vi "Add PV - I32 Array.vi"(5 "is read only? (F)":bool, 6 "initial timestamp":timestamp, 7 "PV name":string, 8 "error in (no error)":errorcluster, 9 "fields":T1, 10 "initial value":i32[](array[numeric]), 11 "Server in":refnum<class "Server.lvclass">) -> (0 "error out":errorcluster, 3 "Server out":refnum<class "Server.lvclass">)   [LabVIEW 2020, in "PV Access.lvlib" / "PVA Server.lvlib" / "Server.lvclass"]
uses:
  Server.lvclass
  PV Data/Value Fields.ctl
  PV Data/NT Scalar (Numeric)/NT Scalar (Numeric).lvclass
  C:/Users/eyw68381/source/repos/pvaccess-labview/labview/source/PV Data/Base/Base.lvclass
  PV Data/NT Scalar (Numeric)/Create - I32 Array.vi
  Source/Source.lvclass
  PV Data/PV Data.lvlib
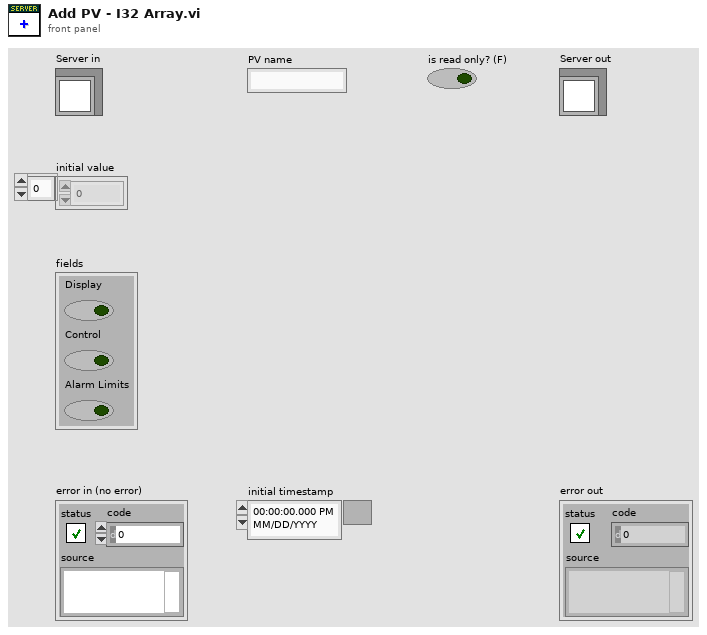
[diagram p1: front panel]
types:
  T1 = typedef "PV Access.lvlib/PV Data.lvlib/Value Fields.ctl" = cluster{"Display":bool, "Control":bool, "Alarm Limits":bool}
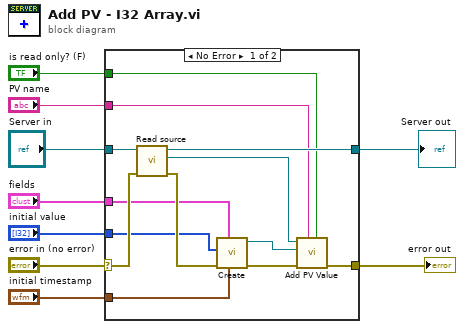
[diagram p0: block diagram]
diagram:
  n1 = case shown="No Error" "error in (no error)" {
    selector: "error in (no error)" -> [w18 w24]
    tunnel: [w17 w24] -> w8
    tunnel: [w21 w23] -> w6
    tunnel: "Server in" -> [w22 w23]
    tunnel: "PV name" -> [w19 _]
    tunnel: "initial value" -> [w13 _]
    tunnel: "fields" -> [w12 _]
    tunnel: "initial timestamp" -> [w11 _]
    tunnel: "is read only? (F)" -> [w10 _]
    frame No Error {
      n2 = call "Read source.vi"("error in (no error)"=w18, "Server in"=w22) -> ("error out"=w16:errorcluster, "Source"=w20:refnum<class "Source.lvclass">, "Server out"=w21:refnum<class "Server.lvclass">)  [unwired: 7 in]
      n3 = call-poly "Create.vi"("timestamp"=w11, "fields"=w12, "error in (no error)"=w16, "value"=w13) -> ("error out"=w15:errorcluster, "NT Scalar (Numeric) out"=w14:refnum<class "NT Scalar (Numeric).lvclass">)  [unwired: 6 in]
      n4 = call "Add PV Value.vi"("is read only? (F)"=w10, "PV name"=w19, "error in"=w15, "NT Base in"=w14, "Source in"=w20) -> ("error out"=w17:errorcluster)  [unwired: 4 in, 2 out]
    }
    frame Error {
    }
  }
  "error out" <- w8
  "Server out" <- w6
